vi "Add Element in Array Altitude Guidance.vi"(8 "error in (no error)":errorcluster, 10 "Guidance In":refnum<class "Guidance.lvclass">, 11 "Vessel in":refnum<class "Vessel.lvclass">) -> (0 "error out":errorcluster, 3 "Vessel out":refnum<class "Vessel.lvclass">)   [LabVIEW 2014, in "Vessel.lvclass"]
uses:
  Vessel.lvclass
  Guidance/Guidance.lvclass
  Vessel.lvclass/Vessel.ctl
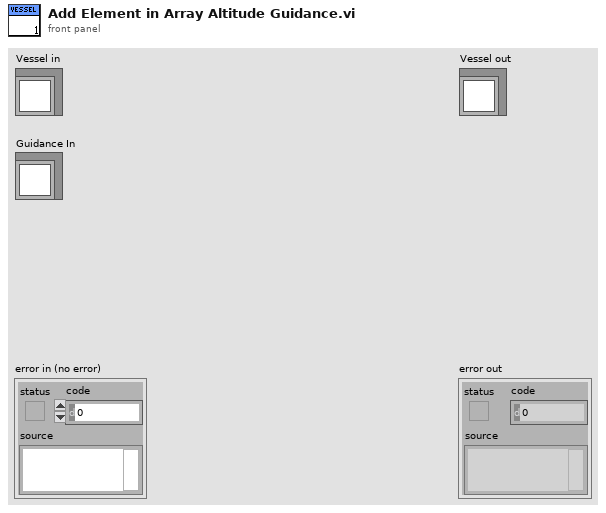
[diagram p1: front panel]
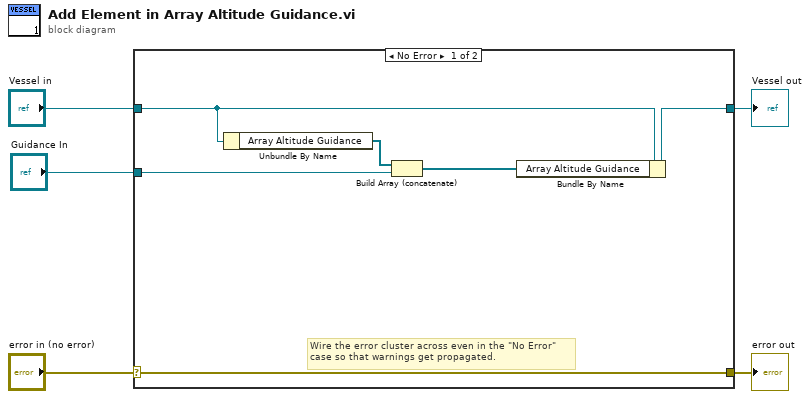
[diagram p0: block diagram]
diagram:
  n1 = case shown="No Error" "error in (no error)" {
    selector: "error in (no error)" -> [w11 w13]
    tunnel: [w11 w13] -> w4
    tunnel: [w7 w12] -> w2
    tunnel: "Vessel in" -> [w8 w12]
    tunnel: "Guidance In" -> [w9 _]
    frame No Error {
      # "Wire the error cluster across even in the \"No Error\"\ncase so that warnings get propagated."
      n2 = Unbundle By Name(w8) -> ("Array Altitude Guidance"=w10:refnum<class "Guidance.lvclass">[])
      n3 = Build Array (concatenate)(w10, w9) -> (w6:refnum<class "Guidance.lvclass">[])
      n4 = Bundle By Name(cluster=w8, "Array Altitude Guidance"=w6) -> (w7:refnum<class "Vessel.lvclass">)
    }
    frame Error {
    }
  }
  "error out" <- w4
  "Vessel out" <- w2
